vi "ZeitabhängigeTXTerstellen.vi"(10 "Signal index to display":i32, 11 "path":path) -> (3 "Path":path)   [LabVIEW 2023]
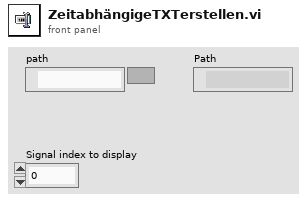
[diagram p1: front panel]
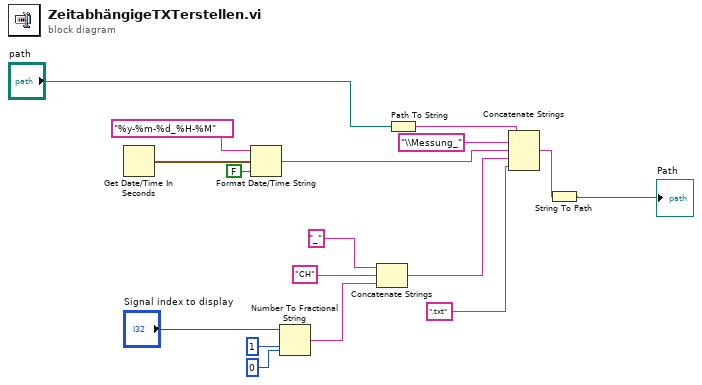
[diagram p0: block diagram]
diagram:
  n1 = Get Date/Time In Seconds() -> (seconds since 1Jan1904=w9:timestamp)
  n2 = Format Date/Time String(time format string (%c)="%y-%m-%d_%H-%M", seconds (now)=w9, UTC format=FALSE) -> (date/time string=w6:string)
  n3 = Number To Fractional String(number="Signal index to display", width (-)=i16 1, precision (6)=i16 0) -> (F-format string=w3:string)  [unwired: 1 in]
  n4 = Concatenate Strings("_" ("string"), "CH" ("string"), w3) -> (w4:string)
  n5 = Path To String(path="path") -> (string=w15:string)
  n6 = Concatenate Strings(w15, "\\Messung_" ("string"), w6, w4, ".txt" ("element")) -> (w14:string)
  n7 = String To Path(string=w14) -> (path=→"Path":path)
